vi "TDMS Write Final.vi"() -> ()   [LabVIEW 2021]
panel:
  in  "Name or path":string
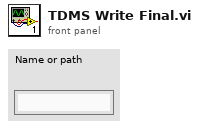
[diagram p1: front panel]
types:
  T1 = enum16{"open", "open or create", "create or replace", "create", "open (read-only)"}
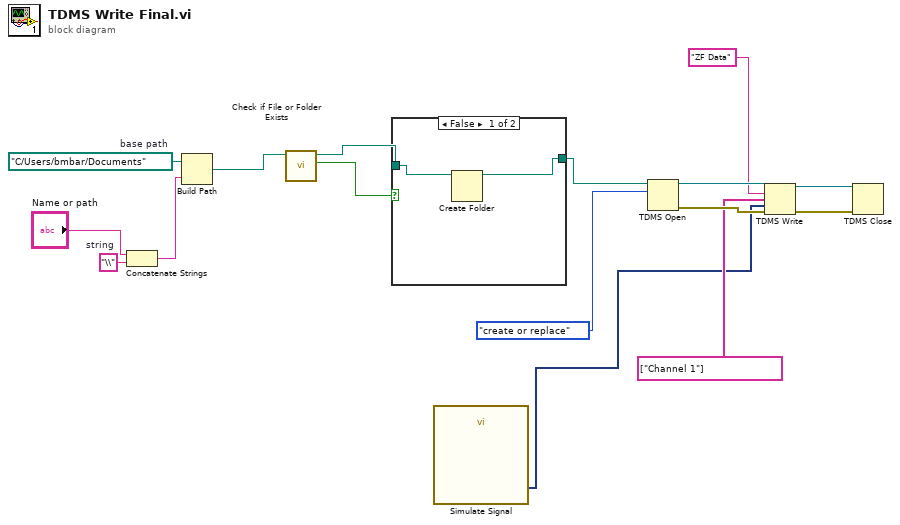
[diagram p0: block diagram]
diagram:
  w12 = "\\"  # string
  w15 = path "C:/Users/bmbar/Documents"  # base path
  n1 = Concatenate Strings "Concatenate Strings"("Name or path", w12) -> (w10:string)
  n2 = Build Path(base path=w15, name or relative path=w10) -> (appended path=w16:path)
  n3 = call <vilib>:"Check if File or Folder Exists.vi"("path"=w16) -> ("file or folder exists?"=w13:bool, "dup path"=w14:path)  [unwired: 8 in, 1 out]
  n4 = case shown="False" w13 {
    tunnel: w14 -> [w18 w19]
    tunnel: [w17 w19] -> w5
    frame False {
      n5 = Create Folder(path (use dialog)=w18) -> (created path=w17:path)  [unwired: 2 in, 2 out]
    }
    frame True {
    }
  }
  n6 = call "Simulate Signal"() -> ("Sine"=w1:dynamicdata)  [unwired: 14 in, 1 out]
  n7 = TDMS Open(10:T1."create or replace" ("operation (0:open)"), 11:w5) -> (0:w7:errorcluster, 3:w9:refnum<k34>)  [unwired: 5 in]
  n8 = TDMS Write(0:w9, 5:"ZF Data" ("group name in (Untitled)"), 7:string[] ["Channel 1"] ("channel name(s) in (Untitled)"), 9:w1, 11:w7) -> (4:w8:refnum<k34>, 15:w6:errorcluster)  [unwired: 1 in, 2 out]
  n9 = TDMS Close(8:w6, 11:w8) -> ()  [unwired: 2 out]
